vi "Xbox Layout.vi"(2 "Joystick Name":string) -> (0 "Center Left":bool, 5 "Arrows":dbl, 6 "Center Right":bool, 7 "A":bool, 8 "Left Button":bool, 9 "B":bool, 10 "Right Button":bool, 11 "X":bool, 12 "L+R Throttles":dbl, 13 "Y":bool, 14 "Left Stick X":dbl, 15 "Left Stick Y":dbl, 16 "Left Stick Touch":bool, 17 "Right Stick X":dbl, 18 "Right Stick Y":dbl, 19 "Right Stick Touch":bool)   [LabVIEW 2013]
doc: "The layout of Buttons and axes from the XBOX 360 Controller"
uses:
  <vilib>/Rock Robotics/WPI/Joystick/WPI_JoystickGetSetRefNum.vi
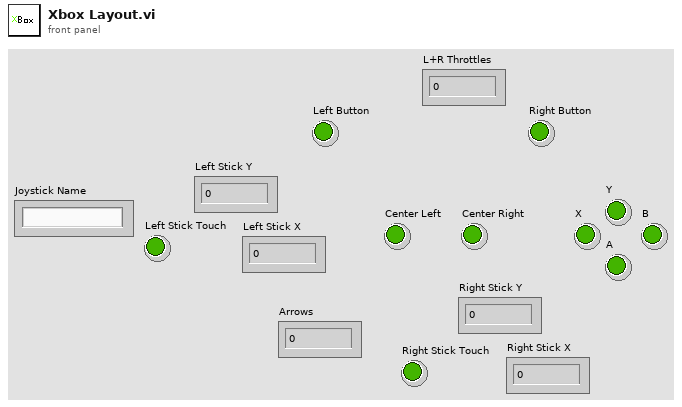
[diagram p1: front panel]
types:
  T1 = typedef "WPI_JoystickDevRef.ctl" = cluster{"Device":T2}
  T2 = typedef "WPI_JoystickDeviceEnum.ctl" = enum16{"USB 1", "USB 2", "USB 3", "USB 4", "Kinect 1", "Kinect 2"}
  T3 = typedef "WPI_JoystickButtonState.ctl" = cluster{"Button 1":bool, "Button 2":bool, "Button 3":bool, "Button 4":bool, "Button 5":bool, "Button 6":bool, "Button 7":bool, "Button 8":bool, "Button 9":bool, "Button 10":bool, "Button 11":bool, "Button 12":bool}
  T4 = cluster{"axis 1 (x)":dbl, "axis 2 (y)":dbl, "axis 3 (throttle)":dbl, "axis 4":dbl, "axis 5":dbl, "axis 6":dbl}
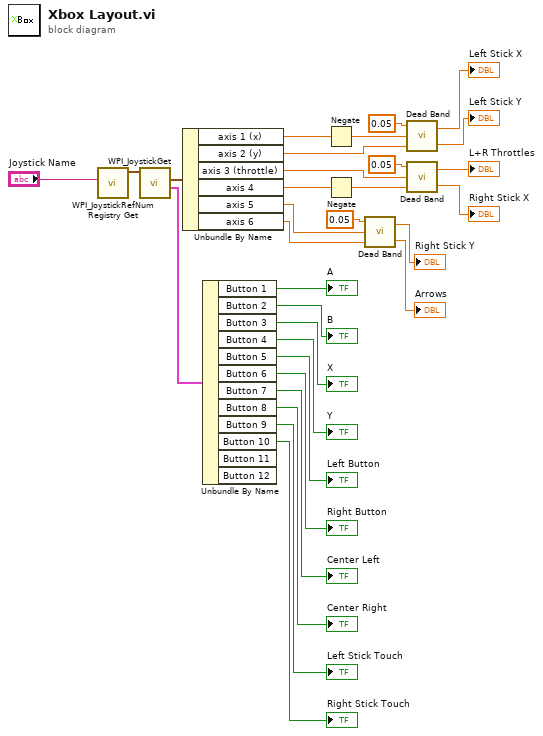
[diagram p0: block diagram]
diagram:
  n1 = call <vilib>:"WPI_JoystickRefNum Registry Get.vi"("refnum name"="Joystick Name") -> ("JoystickDevRef"=w31:T1)  [unwired: 9 in, 1 out]
  n2 = call <vilib>:"WPI_JoystickGet.vi"("JoystickDevRef"=w31) -> ("Buttons"=w29:T3, "Axes"=w28:T4)  [unwired: 4 in, 1 out]
  n3 = Unbundle By Name(w28) -> ("axis 1 (x)"=w27:dbl, "axis 2 (y)"=w9:dbl, "axis 3 (throttle)"=w7:dbl, "axis 4"=w26:dbl, "axis 5"=w3:dbl, "axis 6"=w1:dbl)
  n4 = Unbundle By Name(w29) -> ("Button 1"=→"A":bool, "Button 2"=→"B":bool, "Button 3"=→"X":bool, "Button 4"=→"Y":bool, "Button 5"=→"Left Button":bool, "Button 6"=→"Right Button":bool, "Button 7"=→"Center Left":bool, "Button 8"=→"Center Right":bool, "Button 9"=→"Left Stick Touch":bool, "Button 10"=→"Right Stick Touch":bool)  [unwired: 2 out]
  n5 = Negate(x=w27) -> (-x=w10:dbl)
  n6 = Negate(x=w26) -> (-x=w6:dbl)
  n7 = call "Dead Band.vi"("Axis 2 In"=w1, "Axis 1 In"=w3, "Dead Band"=0.05) -> ("Axis 2 Out"=→"Arrows":dbl, "Axis 1 Out"=→"Right Stick Y":dbl)
  n8 = call "Dead Band.vi"("Axis 2 In"=w9, "Axis 1 In"=w10, "Dead Band"=0.05) -> ("Axis 2 Out"=→"Left Stick Y":dbl, "Axis 1 Out"=→"Left Stick X":dbl)
  n9 = call "Dead Band.vi"("Axis 2 In"=w6, "Axis 1 In"=w7, "Dead Band"=0.05) -> ("Axis 2 Out"=→"Right Stick X":dbl, "Axis 1 Out"=→"L+R Throttles":dbl)
